vi "Control Loop.vi"(11 "Control Loop Cluster":T1) -> (0 "error out":errorcluster)   [LabVIEW 2023, in "RT Main.lvlib"]
uses:
  RT Main.lvlib
  Control Loop Cluster.ctl
  <vilib>/myRIO/Instrument Drivers/Onboard IO/AI/typedefs/AI Reference.ctl
  <vilib>/myRIO/Common/Instrument Driver Framework/Utilities/typedefs/myRIO Generic Hardware Reference.ctl
  <vilib>/myRIO/Common/Instrument Driver Framework/Utilities/typedefs/Hardware Version Enum.ctl
  <vilib>/myRIO/Common/Instrument Driver Framework/Utilities/typedefs/myRIO v1.0 Reference.ctl
  <vilib>/myRIO/Common/Instrument Driver Framework/Utilities/typedefs/Generic FPGA Reference.ctl
  <vilib>/myRIO/Common/Instrument Driver Framework/myRIO v1.0/AI/typedefs/AI Channels List.ctl
  <vilib>/myRIO/Common/Instrument Driver Framework/myRIO v1.0/AI/typedefs/AI Channels Enum.ctl
  <vilib>/myRIO/Common/Instrument Driver Framework/Utilities/typedefs/Analog Scaling Constants List.ctl
  <vilib>/myRIO/Common/Instrument Driver Framework/Utilities/typedefs/Analog Scaling Constants.ctl
  <vilib>/myRIO/Instrument Drivers/Onboard IO/DIO/typedefs/DIO Reference.ctl
  <vilib>/myRIO/Common/Instrument Driver Framework/myRIO v1.0/DIO/typedefs/DIO Channels List.ctl
  <vilib>/myRIO/Common/Instrument Driver Framework/myRIO v1.0/DIO/typedefs/DIO Channels Enum.ctl
  Data Cluster.ctl
  Hardware Monitoring.ctl
  <vilib>/Platform/TimedLoop/XDataNode/timing_clust.ctl
  <vilib>/Platform/TimedLoop/XDataNode/nitl_modes.ctl
  <vilib>/Platform/TimedLoop/XDataNode/wakeup.ctl
  <vilib>/Platform/TimedLoop/TimeConversion.llb/rt-microseconds-to-rel-time.vi
  <vilib>/platform/TimedLoop/XDataNode/XDataNode.xnode
  <vilib>/Platform/TimedLoop/XDataNode/XDNodeRunTimeDep.lvlib
  <vilib>/myRIO/Instrument Drivers/Onboard IO/AI/AI.lvlib
  <vilib>/myRIO/Instrument Drivers/Onboard IO/DIO/DIO.lvlib
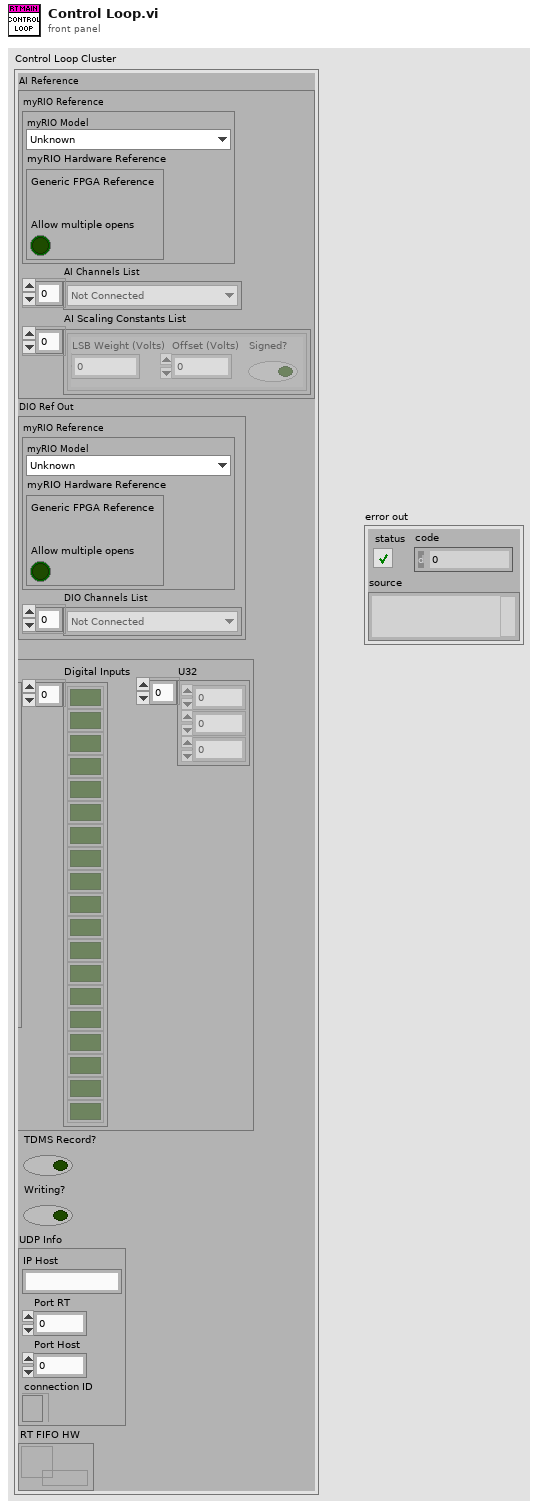
[diagram p1: front panel]
types:
  T1 = typedef "RT Main.lvlib/Control Loop Cluster.ctl" = cluster{"AI Reference":T2, "DIO Reference":T11, "Data Cluster":T14, "TDMS Record?":bool, "Writing?":bool, "UDP Info":cluster{"IP Host":string, "Port RT":u16, "Port Host":u16, "connection ID":refnum<k16>}, "RT FIFO HW":refnum<k33>}
  T2 = typedef "AI.lvlib/AI Reference.ctl" = cluster{"myRIO Reference":T3, "AI Channels List":T7, "AI Scaling Constants List":T9}
  T3 = typedef "myRIO Generic Hardware Reference.ctl" = cluster{"myRIO Model":T4, "myRIO Hardware Reference":T5}
  T4 = typedef "Hardware Version Enum.ctl" = enum16{"Unknown", "myRIO-1900", "myRIO-1950", "roboRIO", "NI ELVIS RIO CM", "ELVIS III"}
  T5 = typedef "myRIO v1.0 Reference.ctl" = cluster{"Generic FPGA Reference":T6, "Allow multiple opens":bool}
  T6 = typedef "Generic FPGA Reference.ctl" = refnum<k20>
  T7 = typedef "AI Channels List.ctl" = T8[]
  T8 = typedef "AI Channels Enum.ctl" = enum16{"Not Connected", "AudioIn/Left", "AudioIn/Right", "C/AI0", "C/AI1", "A/AI0", "A/AI1", "A/AI2", "A/AI3", "A/AI4", "A/AI5", "A/AI6", "A/AI7", "B/AI0", "B/AI1", "B/AI2", "B/AI3", "B/AI4", "B/AI5", "B/AI6", "B/AI7", "AI/AI0", "AI/AI1", "AI/AI2", "AI/AI3", "A/AI0 (DIFF)", "A/AI1 (DIFF)", "A/AI2 (DIFF)", "A/AI3 (DIFF)", "B/AI0 (DIFF)", "B/AI1 (DIFF)", "B/AI2 (DIFF)", "B/AI3 (DIFF)"}
  T9 = typedef "Analog Scaling Constants List.ctl" = T10[]
  T10 = typedef "Analog Scaling Constants.ctl" = cluster{"LSB Weight (Volts)":dbl, "Offset (Volts)":dbl, "Signed?":bool}
  T11 = typedef "DIO.lvlib/DIO Reference.ctl" = cluster{"myRIO Reference":T3, "DIO Channels List":T12}
  T12 = typedef "DIO Channels List.ctl" = T13[]
  T13 = typedef "DIO Channels Enum.ctl" = enum16{"Not Connected", "C/DIO0", "C/DIO1", "C/DIO2", "C/DIO3", "C/DIO4", "C/DIO5", "C/DIO6", "C/DIO7", "A/DIO0", "A/DIO1", "A/DIO2", "A/DIO3", "A/DIO4", "A/DIO5", "A/DIO6", "A/DIO7", "A/DIO8", "A/DIO9", "A/DIO10", "A/DIO11", "A/DIO12", "A/DIO13", "A/DIO14", "A/DIO15", "A/DIO16", "A/DIO17", "A/DIO18", "A/DIO19", "B/DIO0", "B/DIO1", "B/DIO2", "B/DIO3", "B/DIO4", "B/DIO5", "B/DIO6", "B/DIO7", "B/DIO8", "B/DIO9", "B/DIO10", "B/DIO11", "B/DIO12", "B/DIO13", "B/DIO14", "B/DIO15", "B/DIO16", "B/DIO17", "B/DIO18", "B/DIO19", "LED0", "LED1", "LED2", "LED3", "Button0", "DIO/DIO0", "DIO/DIO1", "DIO/DIO2", "DIO/DIO3", "DIO/DIO4", "DIO/DIO5", "DIO/DIO6", "DIO/DIO7", "DIO/DIO8", "DIO/DIO9", "SPI/CS0", "SPI/CS1", "SPI/CS2", "SPI/CS3", "LED RADIO (Green)", "LED RADIO (Red)", "LED COMM (Green)", "LED COMM (Red)", "LED MODE (Green)", "LED MODE (Red)"}
  T14 = typedef "RT Main.lvlib/Data Cluster.ctl" = cluster{"Analog Input":dbl[], "Digital Inputs":bool[], "U32":u32[]}
  T15 = typedef "XDNodeRunTimeDep.lvlib/timing_clust.ctl" = cluster{"Expected End [f-1]":u64, "Actual End [f-1]":u64, "Finished Late? [f-1]":bool, "Expected End [i-1]":u64, "Actual End [i-1]":u64, "Finished Late? [i-1]":bool, "Expected Start [i]":u64, "Actual Start [i]":u64, "Expected Start [f]":u64, "Actual Start [f]":u64, "Source Name":string, "Structure Name":string, "Period":i64, "Deadline":i64, "Offset":i64, "Start":i64, "Priority":i32, "Timeout":i32, "Mode":T16, "Wakeup Reason":T17, "Error":errorcluster, "Source Type":string, "Secondary Source Type":string, "Global End Time":u64, "Global Start Time":u64, "Frame Duration":u64, "Iteration Duration":u64, "Assigned CPU":i32, "I/O Scan Engine Mode":u32}
  T16 = typedef "XDNodeRunTimeDep.lvlib/nitl_modes.ctl" = enum32{"No Change", "Process missed periods, maintain original phase", "Discard missed periods, maintain original phase", "Process missed periods, ignore original phase", "Discard missed periods, ignore original phase"}
  T17 = typedef "XDNodeRunTimeDep.lvlib/wakeup.ctl" = enum32{"Normal", "Aborted", "Asynchronous wakeup", "Timing source error", "Timed loop error", "Timeout"}
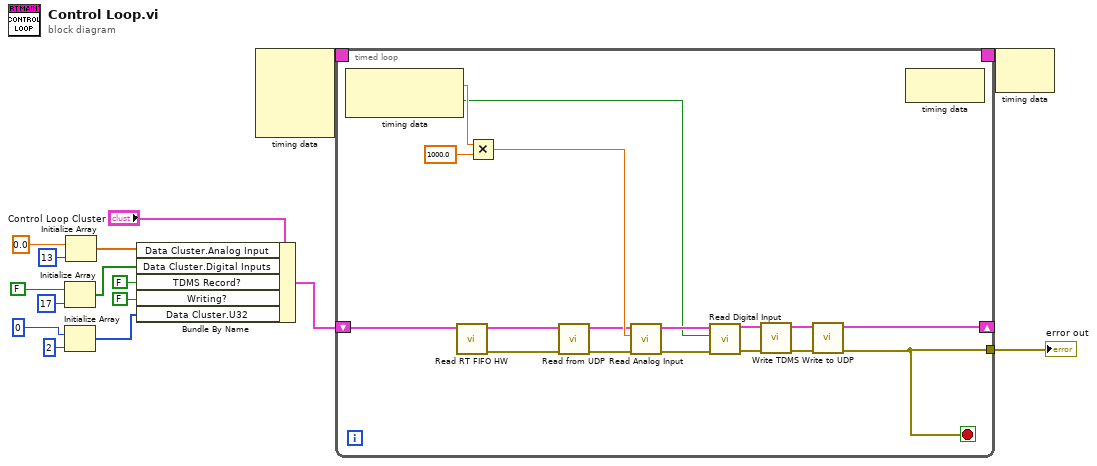
[diagram p0: block diagram]
diagram:
  n1 = Initialize Array(FALSE, 17 ("dimension size")) -> (w6:bool[])
  n2 = Initialize Array(u32 0 ("Numeric"), 2 ("dimension size")) -> (w1:u32[])
  n3 = Initialize Array(0.0 ("element"), 13 ("dimension size")) -> (w12:dbl[])
  n4 = Bundle By Name(cluster="Control Loop Cluster", "Data Cluster.Analog Input"=w12, "Data Cluster.Digital Inputs"=w6, "TDMS Record?"=FALSE, "Writing?"=FALSE, "Data Cluster.U32"=w1) -> (w13:T1)
  n5 = node-c288() -> (w16:T15)  [unwired: 4 in]
  n6 = timed-loop {
    timing: w16 -> [_]
    timing-out: [_] -> w15
    shift-right: [w23] -> _
    shift-left: w13 -> [w19]
    tunnel: [w22] -> w9
    stop <- w22 stop-if-true
    n7 = node-c288() -> (w33:dbl, w24:bool)  [unwired: 1 in]
    n8 = call "Read RT FIFO HW.vi"("Control Loop Cluster"=w19) -> ("error out"=w17:errorcluster, "Control Loop Cluster Out"=w18:T1)  [unwired: 9 in]
    n9 = Multiply(x=w33, y=1000.0) -> (x*y=w32:dbl)
    n10 = call "Read from UDP.vi"("error in"=w17, "Control Loop Cluster"=w18) -> ("error out"=w20:errorcluster, "Control Loop Cluster Out"=w21:T1)  [unwired: 8 in]
    n11 = call "Read Analog Input.vi"("error in"=w20, "Iteration Duration"=w32, "Control Loop Cluster"=w21) -> ("error out"=w29:errorcluster, "Control Loop Cluster Out"=w30:T1)  [unwired: 7 in]
    n12 = call "Read Digital Input.vi"("error in"=w29, "Finish Late"=w24, "Control Loop Cluster"=w30) -> ("error out"=w27:errorcluster, "Control Loop Cluster Out"=w28:T1)  [unwired: 7 in]
    n13 = call "Write TDMS.vi"("error in"=w27, "Control Loop Cluster"=w28) -> ("error out"=w25:errorcluster, "Control Loop Cluster Out"=w26:T1)  [unwired: 8 in]
    n14 = call "Write to UDP.vi"("error in"=w25, "Control Loop Cluster"=w26) -> ("error out"=w22:errorcluster, "Control Loop Cluster Out"=w23:T1)  [unwired: 8 in]
    n15 = node-c288() -> ()  [unwired: 1 in, 1 out]
  }
  "error out" <- w9
  n16 = node-c288(w15) -> ()  [unwired: 1 out]
